vi "Start WiFi.vi"(7 "Retry wait time [ms]":u32=500, 8 "Error In":errorcluster, 10 "TCP Configuration":T5, 11 "LINX Resource":T1) -> (0 "error out":errorcluster, 2 "TCP Config out":T5, 3 "LINX Resource Out":T1)   [LabVIEW 2019, in "LINXx.lvlib"]
doc: "Verify that specified address matches that in board's memory. For DHCP, attempts to reset TCP connection and returns when a valid address is produced."
uses:
  LINXx.lvlib
  <vilib>/MakerHub/LINX/Private/Device/Type Defs/TCP Config.ctl
  <vilib>/MakerHub/LINX/Private/Type Defs/LINX Ref.ctl
  <vilib>/MakerHub/LINX/Private/Type Defs/Platform.ctl
  <vilib>/MakerHub/LINX/Private/Type Defs/Interface.ctl
  <vilib>/MakerHub/LINX/Private/Device/Type Defs/LINX Device Config.ctl
  <vilib>/MakerHub/LINX/Private/Device/Type Defs/Channels.ctl
  <vilib>/Utility/error.llb/DialogType.ctl
  <vilib>/Utility/error.llb/Error Cluster From Error Code.vi
  <vilib>/ErrorRing/Error Ring.xnode
  <vilib>/MakerHub/LINX/Private/Device/Device.lvlib
  <vilib>/MakerHub/LINX/LMH-LINX.lvlib
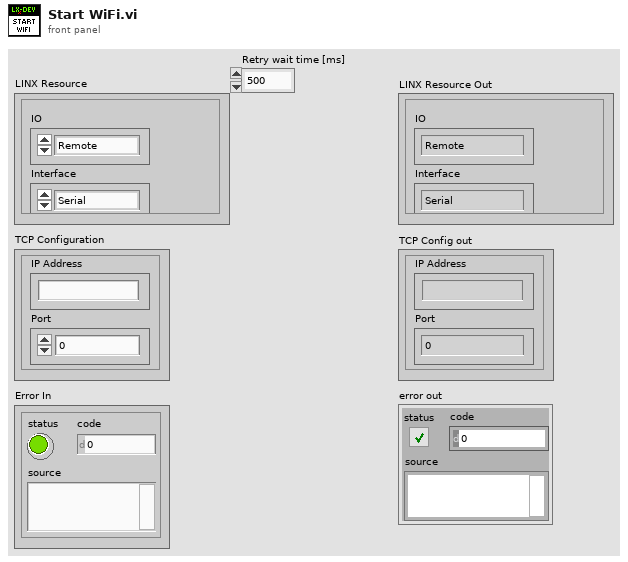
[diagram p1: front panel]
types:
  T1 = typedef "LMH-LINX.lvlib/LINX Ref.ctl" = cluster{"IO":T2, "Interface":T3, "LINX Device Config":T4}
  T2 = typedef "LMH-LINX.lvlib/Platform.ctl" = enum16{"Remote", "Local"}
  T3 = typedef "LMH-LINX.lvlib/Interface.ctl" = enum16{"Serial", "TCP"}
  T4 = typedef "LMH-LINX.lvlib/Device.lvlib/LINX Device Config.ctl" = cluster{"Interface":T3, "COM Port":refnum<visa-resource-name>, "TCP Configuration":T5, "Device Family":u8, "Device ID":u8, "Device Name":string, "TCP Ref":refnum<k5>, "Channels":T6}
  T5 = typedef "LMH-LINX.lvlib/Device.lvlib/TCP Config.ctl" = cluster{"IP Address":string, "Port":u16}
  T6 = typedef "LMH-LINX.lvlib/Channels.ctl" = cluster{"DI":u8[], "DO":u8[], "AI":u8[], "AO":u8[], "PWM":u8[], "QE":u8[], "UART":u8[], "I2C 2":u8[], "SPI":u8[], "CAN":u8[], "Servo":u8[], "AI Ref (V)":dbl, "AI Resolution (Bits)":u8, "AO Ref (V)":dbl, "AO Resolution (Bits)":u8}
  T7 = typedef "DialogType.ctl" = u16
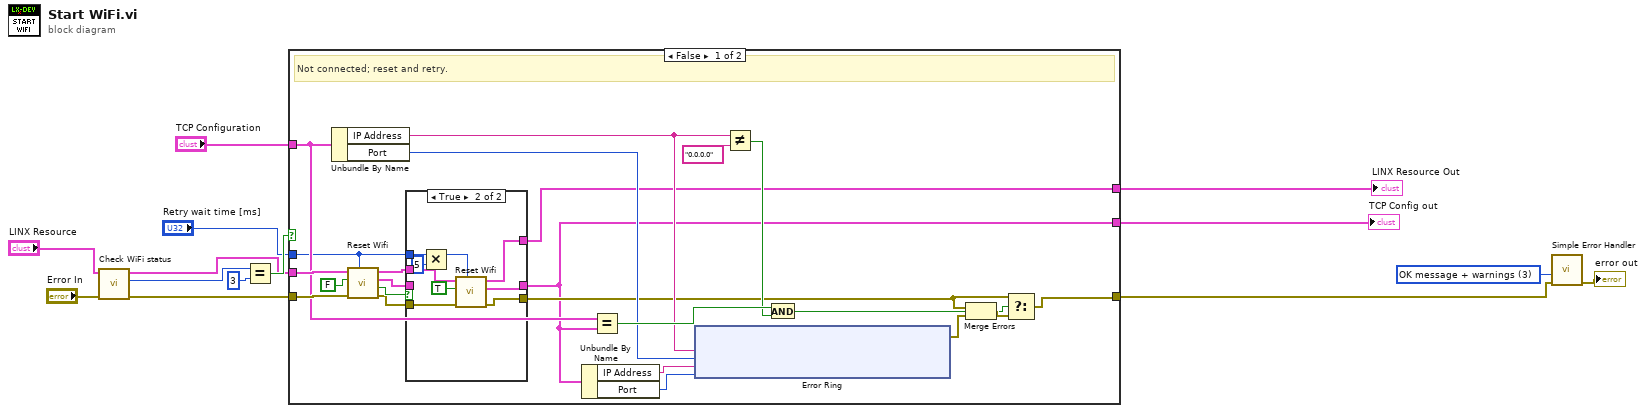
[diagram p0: block diagram]
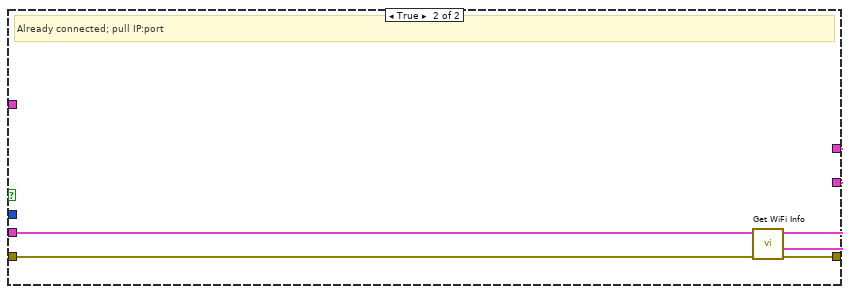
[diagram p3: hidden frame]
diagram:
  w13 = T7 3 items=["no dialog", "OK message", "continue or stop message", "OK message + warnings", "continue/stop + warnings"] ("type of dialog (OK msg:1)")
  n1 = call "Check WiFi status.vi"("Error In"="Error In", "LINX Resource"="LINX Resource") -> ("Error Out"=w9:errorcluster, "WiFi status"=w12:u8, "LINX Resource out"=w8:T1)  [unwired: 7 in]
  n2 = Equal?(x=w12, y=u8 3) -> (x = y?=w10:bool)
  n3 = case shown="False" w10 {
    tunnel: w9 -> [w36 w64]
    tunnel: w8 -> [w37 w63]
    tunnel: [w23 w62] -> w1
    tunnel: "TCP Configuration" -> [w24 _]
    tunnel: "Retry wait time [ms]" -> [w21 _]
    tunnel: [w15 w61] -> w3
    tunnel: [w19 w60] -> w2
    frame False {
      # "Not connected; reset and retry."
      n4 = Unbundle By Name(w24) -> ("IP Address"=w30:string, "Port"=w31:u16)
      n5 = call "Reset Wifi.vi"("Retry wait time [ms]"=w21, "error in (no error)"=w36, "Hard Reset?"=FALSE, "LINX Resource"=w37) -> ("error out"=w18:errorcluster, "Connected?"=w22:bool, "TCP Config"=w16:T5, "LINX Resource Out"=w20:T1)  [unwired: 4 in]
      n6 = case shown="True" w22 {
        tunnel: w21 -> [_ w49]
        tunnel: w20 -> [w39 w48]
        tunnel: [w39 w47] -> w19
        tunnel: w18 -> [w40 w46]
        tunnel: [w40 w45] -> w17
        tunnel: w16 -> [w38 _]
        tunnel: [w38 w43] -> w15
        frame False {
        }
        frame True {
          n7 = Multiply(x=w49, y=u32 5) -> (x*y=w42:u32)
          n8 = call "Reset Wifi.vi"("Retry wait time [ms]"=w42, "error in (no error)"=w46, "Hard Reset?"=TRUE, "LINX Resource"=w48) -> ("error out"=w45:errorcluster, "TCP Config"=w43:T5, "LINX Resource Out"=w47:T1)  [unwired: 4 in, 1 out]
        }
      }
      n9 = Unbundle By Name(w15) -> ("IP Address"=w26:string, "Port"=w25:u16)
      n10 = Equal?(x=w24, y=w15) -> (x = y?=w32:bool)
      n11 = xnode "Error Ring"("parameter 0"=w30, "parameter 1"=w31, "parameter 2"=w26, "parameter 3"=w25) -> ("error out"=w34:errorcluster)
      n12 = Not Equal?(x=w30, y="0.0.0.0") -> (x != y?=w27:bool)
      n13 = And(x=w32, y=w27) -> (x .and. y?=w28:bool)
      n14 = Merge Errors(w17, w34) -> (w33:errorcluster)
      n15 = Select(t=w17, s=w28, f=w33) -> (s? t:f=w23:errorcluster)
    }
    frame True {
      # "Already connected; pull IP:port"
      n16 = call "Get WiFi Info.vi"("Error In"=w64, "LINX Resource"=w63) -> ("Error Out"=w62:errorcluster, "TCP Config"=w61:T5, "LINX Resource Out"=w60:T1)  [unwired: 6 in, 1 out]
    }
  }
  "TCP Config out" <- w3
  "LINX Resource Out" <- w2
  n17 = call <vilib>:"Simple Error Handler.vi"("type of dialog (OK msg:1)"=w13, "error in (no error)"=w1) -> ("error out"=→"error out":errorcluster)  [unwired: 3 in, 4 out]
